vi "swbomb.vi"() -> (3 "BOMB":bool)   [LabVIEW 2016]
panel:
  out "data":timestamp
  out "current time":timestamp
  out "Numeric":i32
  out "Lastdate":timestamp
  out "t":string
  in  "Data limite":timestamp=timestamp(3689573984.708 s since 1904-01-01)
  # "salva come default!"
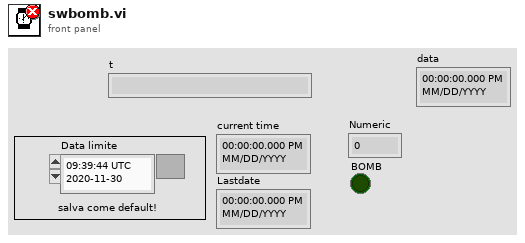
[diagram p1: front panel]
types:
  T1 = enum16{"open", "replace", "create", "open or create", "replace or create", "replace or create with confirmation"}
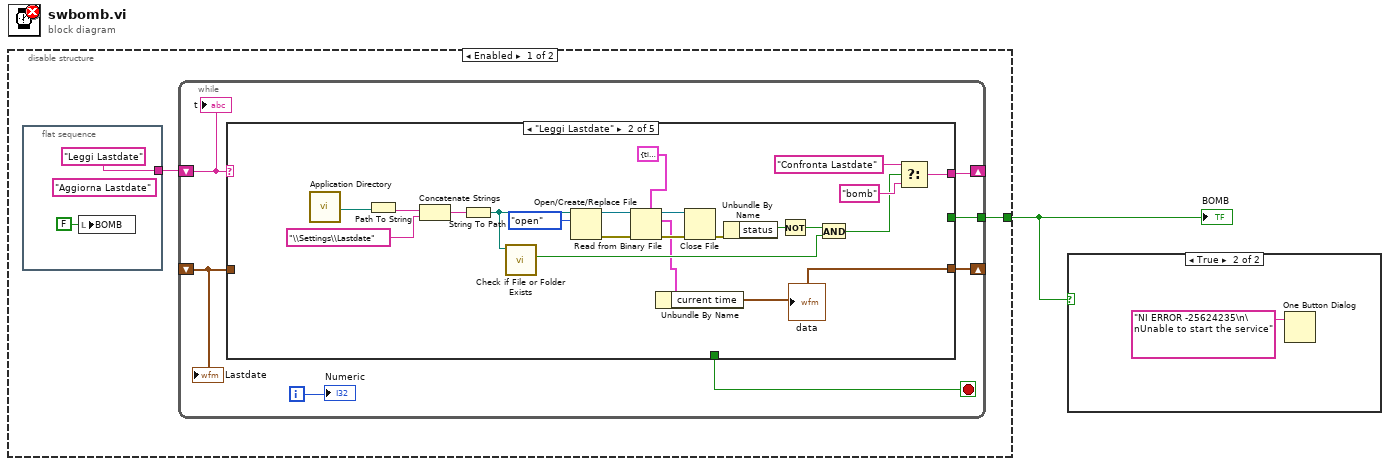
[diagram p0: block diagram]
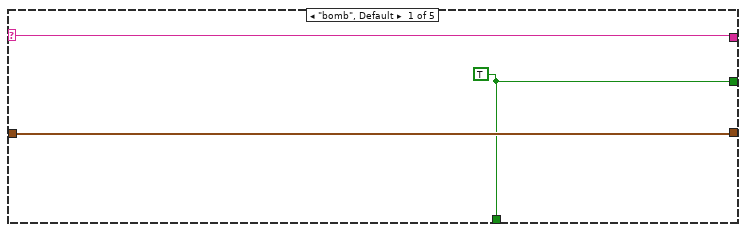
[diagram p3: hidden frame]
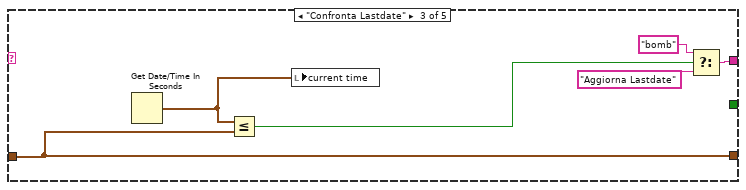
[diagram p4: hidden frame]
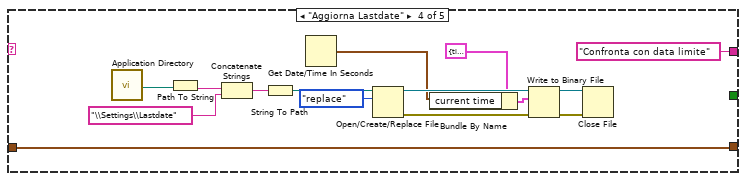
[diagram p5: hidden frame]
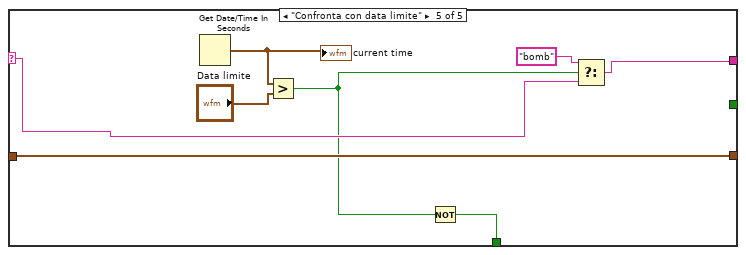
[diagram p6: hidden frame]
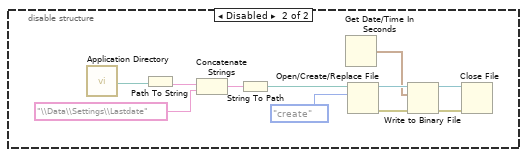
[diagram p7: hidden frame]
diagram:
  n1 = disable-structure shown="Enabled" {
    disable-tunnel: [w2 _] -> w1
    frame Enabled {
      n2 = flat-sequence {
        tunnel: ["Leggi Lastdate"] -> w3
        frame #0 {
          (unwired) "Aggiorna Lastdate"
          n3 = local write "BOMB"(FALSE ("x > y?")) -> ()
        }
      }
      n4 = while {
        shift-right: [w11] -> _
        shift-left: w3 -> [w12]
        shift-right: [w10] -> _
        shift-left: _ -> [w9]
        tunnel: [w6] -> w2
        i -> [w8]
        stop <- w7 stop-if-true
        n5 = case shown="\"Leggi Lastdate\"" w12 {
          selector: w12 -> [w15 _ _ _ w62]
          tunnel: [w15 w26 w40 "Confronta con data limite" ("t") w61] -> w11
          tunnel: [w14 w16 w38 w48 w60] -> w10
          tunnel: w9 -> [w14 _ w38 w48 w60]
          tunnel: [w13 _ _ _ w58] -> w7
          tunnel: [w13 _ _ _ _] -> w6
          frame "bomb", Default {
            w13 = TRUE ("x > y?")
          }
          frame "Leggi Lastdate" {
            n6 = call <vilib>:"Application Directory.vi"() -> ("Application Directory"=w36:path)
            n7 = Path To String(path=w36) -> (string=w35:string)
            n8 = Concatenate Strings(w35, "\\Settings\\Lastdate" ("string")) -> (w33:string)
            n9 = String To Path(string=w33) -> (path=w32:path)
            n10 = call <vilib>:"Check if File or Folder Exists.vi"("path"=w32) -> ("file or folder exists?"=w22:bool)  [unwired: 8 in, 2 out]
            n11 = Open/Create/Replace File(file path (use dialog)=w32, operation (0:open)=T1."open") -> (refnum out=w31:refnum<file>, error out=w30:errorcluster)  [unwired: 4 in, 1 out]
            n12 = Read from Binary File(5:cluster{"current time":timestamp} {"current time"=timestamp(0 s since 1904-01-01)}, 8:w30, 11:w31) -> (0:w28:errorcluster, 2:w17:cluster{"current time":timestamp}, 3:w29:refnum<file>)  [unwired: 3 in, 1 out]
            n13 = Unbundle By Name(w17) -> ("current time"=w16:timestamp)
            "data" <- w16
            n14 = Close File(refnum=w29, error in=w28) -> (error out=w24:errorcluster)  [unwired: 1 out]
            n15 = Unbundle By Name(w24) -> ("status"=w23:bool)
            n16 = Not(x=w23) -> (.not. x?=w20:bool)
            n17 = And(x=w20, y=w22) -> (x .and. y?=w21:bool)
            n18 = Select(t="Confronta Lastdate", s=w21, f="bomb") -> (s? t:f=w26:string)
          }
          frame "Confronta Lastdate" {
            n19 = Get Date/Time In Seconds() -> (seconds since 1Jan1904=w37:timestamp)
            n20 = Less Or Equal?(x=w37, y=w38) -> (x <= y?=w42:bool)
            n21 = local write "current time"(w37) -> ()
            n22 = Select(t="bomb", s=w42, f="Aggiorna Lastdate") -> (s? t:f=w40:string)
          }
          frame "Aggiorna Lastdate" {
            n23 = call <vilib>:"Application Directory.vi"() -> ("Application Directory"=w57:path)
            n24 = Path To String(path=w57) -> (string=w56:string)
            n25 = Concatenate Strings(w56, "\\Settings\\Lastdate" ("string")) -> (w54:string)
            n26 = String To Path(string=w54) -> (path=w53:path)
            n27 = Get Date/Time In Seconds() -> (seconds since 1Jan1904=w44:timestamp)
            n28 = Open/Create/Replace File(file path (use dialog)=w53, operation (0:open)=T1."replace") -> (refnum out=w52:refnum<file>, error out=w51:errorcluster)  [unwired: 4 in, 1 out]
            n29 = Bundle By Name(cluster=cluster{"current time":timestamp} {"current time"=timestamp(0 s since 1904-01-01)}, "current time"=w44) -> (w43:cluster{"current time":timestamp})
            n30 = Write to Binary File(file (use dialog)=w52, data=w43, error in=w51) -> (refnum out=w50:refnum<file>, error out=w49:errorcluster)  [unwired: 3 in, 1 out]
            n31 = Close File(refnum=w50, error in=w49) -> ()  [unwired: 2 out]
          }
          frame "Confronta con data limite" {
            n32 = Get Date/Time In Seconds() -> (seconds since 1Jan1904=w65:timestamp)
            "current time" <- w65
            n33 = Greater?(x=w65, y="Data limite") -> (0:w59:bool)
            n34 = Not(x=w59) -> (.not. x?=w58:bool)
            n35 = Select(t="bomb", s=w59, f=w62) -> (s? t:f=w61:string)
          }
        }
        "t" <- w12
        "Lastdate" <- w9
        "Numeric" <- w8
      }
    }
    frame Disabled {
      n36 = call <vilib>:"Application Directory.vi"() -> ("Application Directory"=w75:path)
      n37 = Path To String(path=w75) -> (string=w74:string)
      n38 = Concatenate Strings(w74, "\\Data\\Settings\\Lastdate" ("string")) -> (w72:string)
      n39 = String To Path(string=w72) -> (path=w71:path)
      n40 = Get Date/Time In Seconds() -> (seconds since 1Jan1904=w66:timestamp)
      n41 = Open/Create/Replace File(file path (use dialog)=w71, operation (0:open)=T1."create") -> (refnum out=w70:refnum<file>, error out=w69:errorcluster)  [unwired: 4 in, 1 out]
      n42 = Write to Binary File(file (use dialog)=w70, data=w66, error in=w69) -> (refnum out=w68:refnum<file>, error out=w67:errorcluster)  [unwired: 3 in, 1 out]
      n43 = Close File(refnum=w68, error in=w67) -> ()  [unwired: 2 out]
    }
  }
  "BOMB" <- w1
  n44 = case shown="True" w1 {
    frame False {
    }
    frame True {
      n45 = One Button Dialog(message="NI ERROR -25624235\n\nUnable to start the service") -> ()  [unwired: 1 in, 1 out]
    }
  }
